vi "Set_parameter.vi"(6 "Delete last CMD":bool, 8 "error in (no error)":errorcluster, 9 "value":dbl, 10 "parameter":string, 11 "Toolbox in":refnum<class "Toolbox.lvclass">) -> (0 "error out":errorcluster, 3 "Toolbox out":refnum<class "Toolbox.lvclass">)   [LabVIEW 2014, in "Driver_interaction.lvlib" / "Toolbox.lvclass"]
uses:
  Toolbox.lvclass
  Toolbox.lvclass/Toolbox.ctl
  _Driver_interaction/_Driver_interaction.lvclass
  Vendor/lib 2p0/FTS 2p0.lvlib
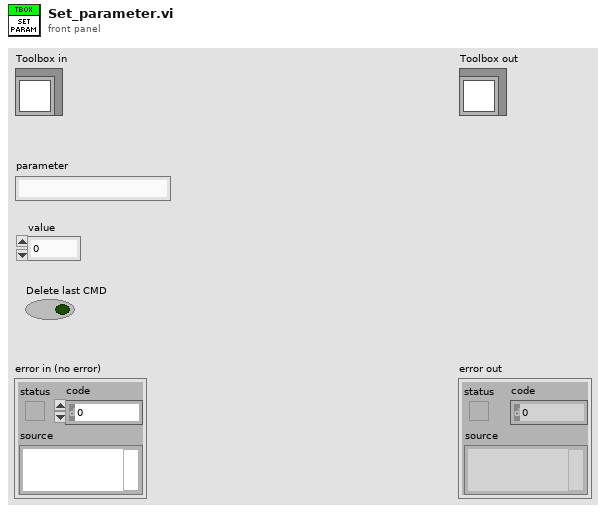
[diagram p1: front panel]
types:
  T1 = typedef "Driver_interaction.lvlib/Toolbox.lvclass/Toolbox_session.ctl" = cluster{"client handle":T2, "URL out":string, "universe_id":i32, "devices_id":i32[]}
  T2 = typedef "LabVIEWHTTPClient.lvlib/ClientHandle.ctl" = refnum<k1>
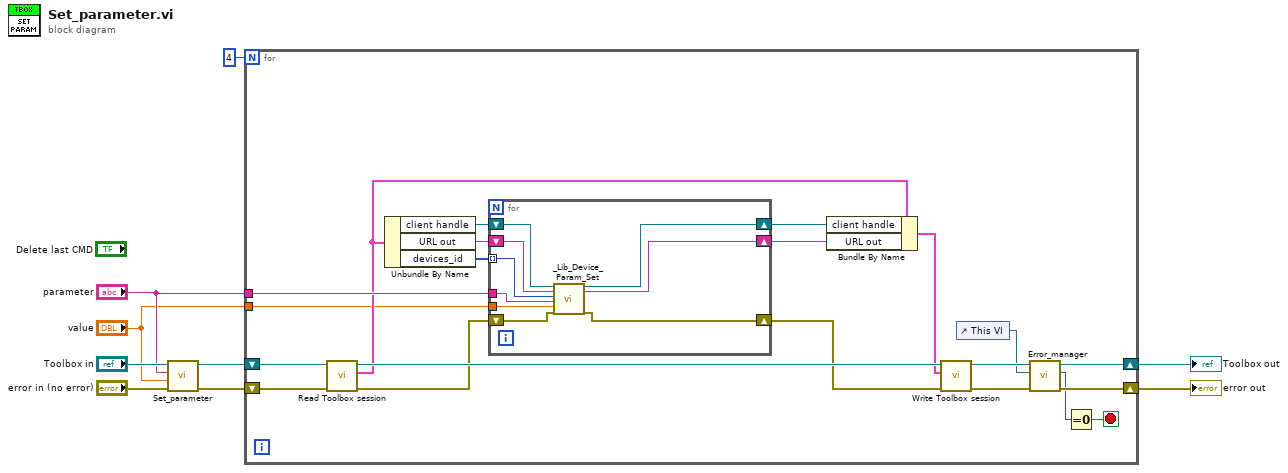
[diagram p0: block diagram]
diagram:
  n1 = call-parent "Set_parameter.vi"("error in (no error)"="error in (no error)", "value"="value", "parameter"="parameter", "_Driver_interaction in"="Toolbox in") -> ("error out"=w4:errorcluster, "_Driver_interaction out"=w3:refnum<class "Toolbox.lvclass">)  [unwired: 6 in]
  n2 = for {
    N: 4 -> [_]
    tunnel: "parameter" -> [w23]
    shift-right: [w15] -> w2
    shift-left: w3 -> [w30]
    shift-right: [w14] -> w1
    shift-left: w4 -> [w28]
    tunnel: "value" -> [w10]
    stop <- w11 stop-if-true
    n3 = call "Read Toolbox session.vi"("error in (no error)"=w28, "Toolbox in"=w30) -> ("error out"=w27:errorcluster, "Toolbox session"=w22:T1, "Toolbox out"=w29:refnum<class "Toolbox.lvclass">)  [unwired: 7 in]
    n4 = Unbundle By Name(w22) -> ("client handle"=w25:T2, "URL out"=w24:string, "devices_id"=w18:i32[])
    n5 = for {
      tunnel: w23 -> [w36]
      shift-right: [w32] -> w26
      shift-left: w27 -> [w35]
      shift-right: [w34] -> w21
      shift-left: w25 -> [w39]
      shift-right: [w33] -> w20
      shift-left: w24 -> [w38]
      tunnel: w18 -> [w37] mode=indexing
      tunnel: w10 -> [w31]
      n6 = call "_Lib_Device_Param_Set.vi"("client handle"=w39, "URL"=w38, "params.device_id"=w37, "params.pid"=w36, "params.value"=w31, "error in (no error)"=w35) -> ("client handle out"=w34:T2, "URL out"=w33:string, "error out"=w32:errorcluster)  [unwired: 11 in]
    }
    n7 = Bundle By Name(cluster=w22, "client handle"=w21, "URL out"=w20) -> (w19:T1)
    n8 = call "Write Toolbox session.vi"("error in (no error)"=w26, "Toolbox session"=w19, "Toolbox in"=w29) -> ("error out"=w17:errorcluster, "Toolbox out"=w16:refnum<class "Toolbox.lvclass">)  [unwired: 7 in]
    n9 = control-ref of="This VI"() -> (w13:refnum<vi>)
    n10 = call-dynamic "Error_manager.vi"("error in (no error)"=w17, "Caller VI"=w13, "Toolbox in"=w16) -> ("error out"=w14:errorcluster, "code"=w12:i32, "Toolbox out"=w15:refnum<class "Toolbox.lvclass">)  [unwired: 4 in, 2 out]
    n11 = Equal To 0?(x=w12) -> (x = 0?=w11:bool)
  }
  "error out" <- w1
  "Toolbox out" <- w2
